vi "Not in the library.vi"() -> ()   [LabVIEW 2015]
uses:
  colors.ctl
  Circle cluster.ctl
  Circle Library.lvlib
panel:
  out "output cluster":T1
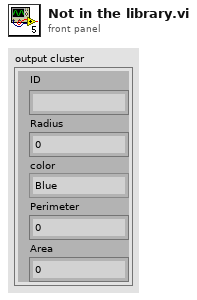
[diagram p1: front panel]
types:
  T1 = typedef "Circle Library.lvlib/Circle cluster.ctl" = cluster{"ID":string, "Radius":dbl, "color":T2, "Perimeter":dbl, "Area":dbl}
  T2 = typedef "colors.ctl" = enum16{"Blue", "Red", "Green", "Yellow"}
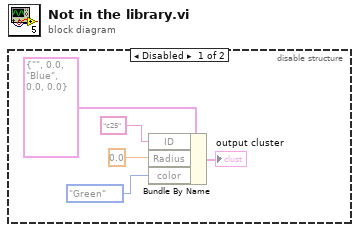
[diagram p0: block diagram]
diagram:
  n1 = disable-structure shown="Disabled" {
    frame Disabled {
      n2 = Bundle By Name(cluster=T1 {"ID"="", "Radius"=0.0, "color"=enum."Blue", "Perimeter"=0.0, "Area"=0.0} ("Circle"), "ID"="c25", "Radius"=0.0, "color"=colors."Green") -> (→"output cluster":T1)
    }
    frame Enabled {
    }
  }
